vi "NI VeriStand - Rename Custom Device Item.vi"(7 "Force Rename? (F)":bool, 8 "error in (no error)":errorcluster, 10 "New Name":string, 11 "Item Ref in":T1 format="%.0x") -> (0 "error out":errorcluster, 2 "Request invalid?":bool, 3 "Item Ref out":T1 format="%.0x")   [LabVIEW 2020, in "Custom Device Offline API.lvlib"]
uses:
  <vilib>/NI VeriStand/Custom Device Offline API/Custom Device Offline API.lvlib
  <vilib>/NI VeriStand/Custom Device API/Custom Device Item Ref.ctl
  NationalInstruments.VeriStand.SystemDefinitionAPI
  <vilib>/NI VeriStand/Custom Device API/Custom Device API.lvlib
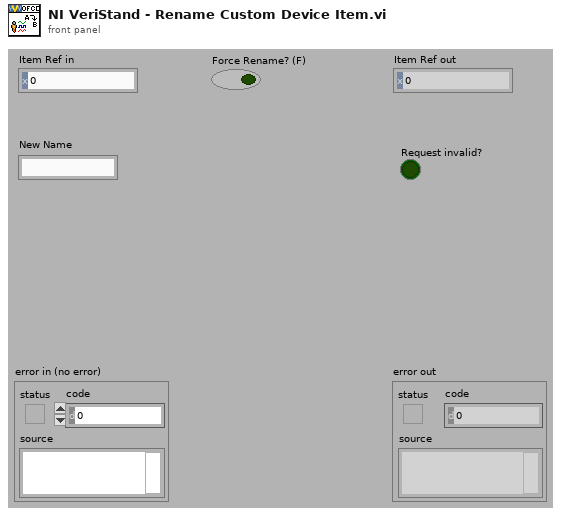
[diagram p1: front panel]
types:
  T1 = typedef "Custom Device API.lvlib/Custom Device Item Ref.ctl" = u64
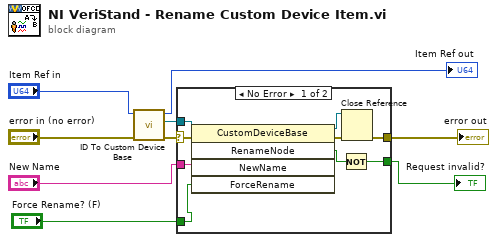
[diagram p0: block diagram]
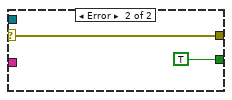
[diagram p2: hidden frame]
diagram:
  n1 = call <vilib>:"ID To Custom Device Base.vi"("error in (no error)"="error in (no error)", "ID in"="Item Ref in") -> ("error out"=w2:errorcluster, "BaseNode"=w6:refnum<k24>, "ID out"=→"Item Ref out":u64)  [unwired: 7 in]
  n2 = case shown="No Error" w2 {
    selector: w2 -> [w11 w20]
    tunnel: w6 -> [w18 _]
    tunnel: "New Name" -> [w17 _]
    tunnel: [w13 w20] -> w4
    tunnel: [w12 TRUE] -> w3
    tunnel: "Force Rename? (F)" -> [w10 _]
    frame No Error {
      n3 = invoke class="CustomDeviceBase" method="RenameNode"(reference=w18, error in=w11, "NewName"=w17, "ForceRename"=w10) -> (reference out=w14:refnum<k24>, error out=w15:errorcluster, "RenameNode"=w16:bool)  [unwired: 1 in, 2 out]
      n4 = Not(x=w16) -> (.not. x?=w12:bool)
      n5 = Close Reference(reference=w14, error in (no error)=w15) -> (error out=w13:errorcluster)
    }
    frame Error {
    }
  }
  "error out" <- w4
  "Request invalid?" <- w3
